vi "Edit DPID.vi"(8 "error in (no error)":errorcluster, 11 "Node Ptr":u64 format="%.0x") -> (0 "error out":errorcluster)   [LabVIEW 2015, in "Diagnostics Addon System Explorer.lvlib"]
uses:
  Diagnostics Addon System Explorer.lvlib
  <vilib>/NI Veristand/Custom Device Tools/Custom Device Utility Library/Search Direction.ctl
  Types/FG.Action.ctl
  SubVIs/ID.FG.vi
  SubVIs/Signals.Get.vi
  SubVIs/Type.FG.vi
  SubVIs/Frame.Convert.Name.vi
  SubVIs/Signal.FG.vi
  Shared/SubVIs/Constants.vi
  <vilib>/NI/NI VeriStand Advanced SysDef API/SysDef API/SysDef.Property.Set.vi
  <vilib>/NI/NI VeriStand Advanced SysDef API/_SubVIs/SysDef.Property.Set.U32.vi
  <vilib>/NI Veristand/Custom Device API/NI VeriStand - Get Item Property.vi
  <vilib>/NI Veristand/Custom Device API/Get Item Property (U32).vi
  <vilib>/NI/NI VeriStand Advanced SysDef API/_SubVIs/SysDef.Property.Set.U32.Array.vi
  <vilib>/NI Veristand/Custom Device API/Get Item Property (U32 Array).vi
  <vilib>/NI Veristand/Custom Device Tools/Custom Device Utility Library/NI VeriStand - Search for Item by GUID.vi
  <vilib>/NI Veristand/Custom Device API/NI VeriStand - Get Item Data.vi
  <vilib>/NI Veristand/Custom Device API/NI VeriStand - Get Item Description.vi
  <vilib>/NI/NI VeriStand Advanced SysDef API/_SubVIs/SysDef.Property.Set.DBL.vi
  <vilib>/NI/NI VeriStand Advanced SysDef API/_SubVIs/SysDef.Property.Set.String.vi
  <vilib>/NI Veristand/Custom Device API/Get Item Property (Double).vi
  <vilib>/NI Veristand/Custom Device API/Get Item Property (String).vi
  <vilib>/NI Veristand/Custom Device API/NI VeriStand - Get Custom Device Channel Data.vi
  <vilib>/NI Veristand/Custom Device Tools/Custom Device Utility Library/Custom Device Utility Library.lvlib
  Shared/Diagnostics Addon Shared.lvlib
  <vilib>/NI Veristand/Custom Device API/Custom Device API.lvlib
panel:
  in  "Tag":string
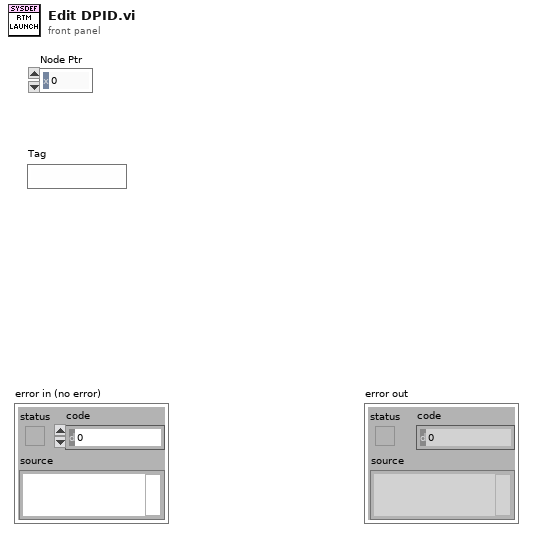
[diagram p1: front panel]
types:
  T1 = typedef "Diagnostics Addon System Explorer.lvlib/FG.Action.ctl" = enum16{"Get", "Set"}
  T2 = typedef "Custom Device Utility Library.lvlib/Search Direction.ctl" = enum16{"Down", "Up"}
  T3 = typedef "Diagnostics Addon Shared.lvlib/DPID.ctl" = cluster{"DPID ID":u8, "Speed":T4, "PIDs":u16[]}
  T4 = typedef "Diagnostics Addon Shared.lvlib/DPID.Rate.ctl" = enum16{"Slow", "Medium", "Fast"}
  T5 = typedef "Custom Device API.lvlib/Custom Device Item Ref.ctl" = u64
  T6 = typedef "Diagnostics Addon System Explorer.lvlib/Frame.Export.ctl" = cluster{"Name":string, "Description":string, "ID":u32, "Signals":T7[]}
  T7 = typedef "Diagnostics Addon Shared.lvlib/Signal.ctl" = cluster{"Start Bit":u32, "Length":u32, "Scaling Factor":dbl, "Scaling Offset":dbl, "Minimum":dbl, "Maximum":dbl, "Data Type":u32, "Byte Order":u32, "Default Value":dbl, "Name":string, "Units":string, "Description":string}
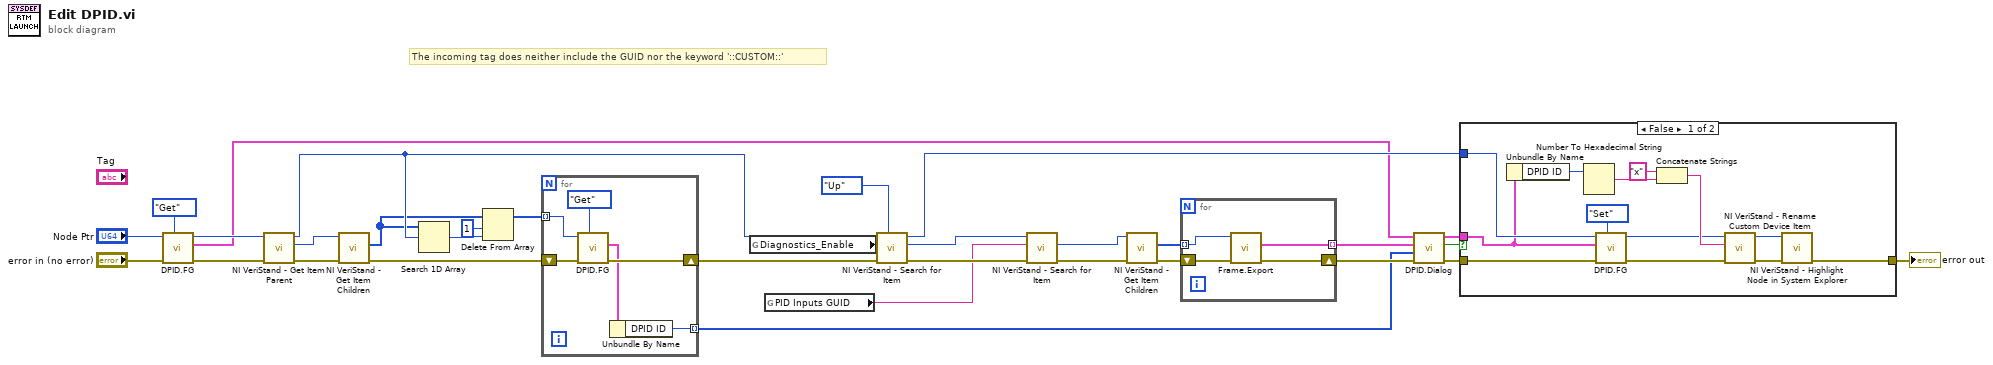
[diagram p0: block diagram]
diagram:
  # "The incoming tag does neither include the GUID nor the keyword '::CUSTOM::'"
  n1 = call "DPID.FG.vi"("Action"=FG.Action."Get", "error in (no error)"="error in (no error)", "Device Item Ref in"="Node Ptr") -> ("error out"=w10:errorcluster, "DPID"=w1:T3, "Device Item Ref out"=w13:T5)  [unwired: 6 in]
  n2 = call <vilib>:"NI VeriStand - Get Item Parent.vi"("error in (no error)"=w10, "Item Ref in"=w13) -> ("error out"=w9:errorcluster, "Parent Ref"=w11:T5, "Item Ref out"=w6:T5)  [unwired: 6 in, 1 out]
  n3 = call <vilib>:"NI VeriStand - Get Item Children.vi"("error in (no error)"=w9, "Item Ref in"=w11) -> ("error out"=w25:errorcluster, "Child Refs"=w5:T5[])  [unwired: 6 in, 2 out]
  n4 = Search 1D Array(1D array=w5, element=w6) -> (index of element=w7:i32)  [unwired: 1 in]
  n5 = Delete From Array(array=w5, length=1, index=w7) -> (array with subset deleted=w4:T5[])  [unwired: 1 out]
  n6 = for {
    tunnel: w4 -> [w38] mode=indexing
    shift-right: [w36] -> w24
    shift-left: w25 -> [w37]
    tunnel: [w34] -> w20 mode=indexing
    n7 = call "DPID.FG.vi"("Action"=FG.Action."Get", "error in (no error)"=w37, "Device Item Ref in"=w38) -> ("error out"=w36:errorcluster, "DPID"=w35:T3)  [unwired: 6 in, 1 out]
    n8 = Unbundle By Name(w35) -> ("DPID ID"=w34:u8)
  }
  n9 = global read "Constants.vi" "Diagnostics_Enable"() -> (w32:string)
  n10 = global read "Constants.vi" "PID Inputs GUID"() -> (w28:string)
  n11 = call-poly <vilib>:"NI VeriStand - Search for Item.vi"("Direction (Down)"=Search_Direction."Up", "error in"=w24, "Item GUID"=w32, "Section Ref in"=w6) -> ("error out"=w29:errorcluster, "Item Ref"=w30:T5, "Section Ref out"=w15:T5)  [unwired: 4 in, 1 out]
  n12 = call-poly <vilib>:"NI VeriStand - Search for Item.vi"("error in"=w29, "Item GUID"=w28, "Section Ref in"=w30) -> ("error out"=w27:errorcluster, "Item Ref"=w26:T5)  [unwired: 5 in, 2 out]
  n13 = call <vilib>:"NI VeriStand - Get Item Children.vi"("error in (no error)"=w27, "Item Ref in"=w26) -> ("error out"=w23:errorcluster, "Child Refs"=w22:T5[])  [unwired: 6 in, 2 out]
  n14 = for {
    tunnel: w22 -> [w42] mode=indexing
    tunnel: [w39] -> w2 mode=indexing
    shift-right: [w40] -> w21
    shift-left: w23 -> [w41]
    n15 = call "Frame.Export.vi"("error in (no error)"=w41, "Item Ref in"=w42) -> ("error out"=w40:errorcluster, "Frame"=w39:T6)  [unwired: 7 in, 1 out]
  }
  n16 = call "DPID.Dialog.vi"("error in (no error)"=w21, "Existing DPIDs"=w20, "Existing PIDs"=w2, "DPID"=w1) -> ("error out"=w17:errorcluster, "Cancel PID?"=w19:bool, "DPID"=w18:T3)  [unwired: 5 in]
  n17 = case shown="False" w19 {
    tunnel: w18 -> [w43 _]
    tunnel: w17 -> [w54 w56]
    tunnel: [w45 w56] -> w16
    tunnel: w15 -> [w55 _]
    frame False {
      n18 = Unbundle By Name(w43) -> ("DPID ID"=w48:u8)
      n19 = Number To Hexadecimal String(2:w48) -> (0:w51:string)  [unwired: 1 in]
      n20 = call "DPID.FG.vi"("Action"=FG.Action."Set", "error in (no error)"=w54, "DPID"=w43, "Device Item Ref in"=w55) -> ("error out"=w50:errorcluster, "Device Item Ref out"=w49:T5)  [unwired: 5 in, 1 out]
      n21 = Concatenate Strings("x" ("element"), w51) -> (w53:string)
      n22 = call <vilib>:"NI VeriStand - Rename Custom Device Item.vi"("error in (no error)"=w50, "New Name"=w53, "Item Ref in"=w49) -> ("error out"=w46:errorcluster, "Item Ref out"=w47:T5)  [unwired: 1 in, 6 out]
      n23 = call <vilib>:"NI VeriStand - Highlight Node in System Explorer.vi"("error in (no error)"=w46, "Item Ref in"=w47) -> ("error out"=w45:errorcluster)  [unwired: 8 in, 1 out]
    }
    frame True {
    }
  }
  "error out" <- w16
